vi "MMF with Identical Structure Element.vi"(7 "signal length":i32, 8 "start index":i32, 9 "operation type":u16(ring) items=["Dilation", "Erosion"], 10 "Structure Element":dbl[](array[numeric]), 11 "Extended X":dbl[](array[numeric])) -> (3 "Filtered X":dbl[](array[numeric]))   [LabVIEW 2020, in "NI_AAL_Filter.lvlib"]
uses:
  <vilib>/Analysis/NI_AAL_Filter.lvlib
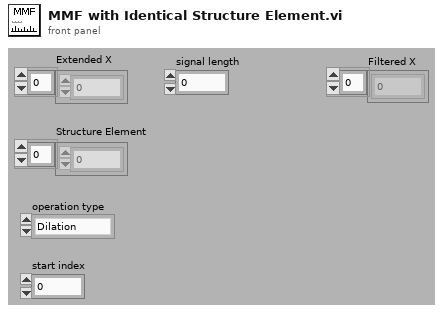
[diagram p1: front panel]
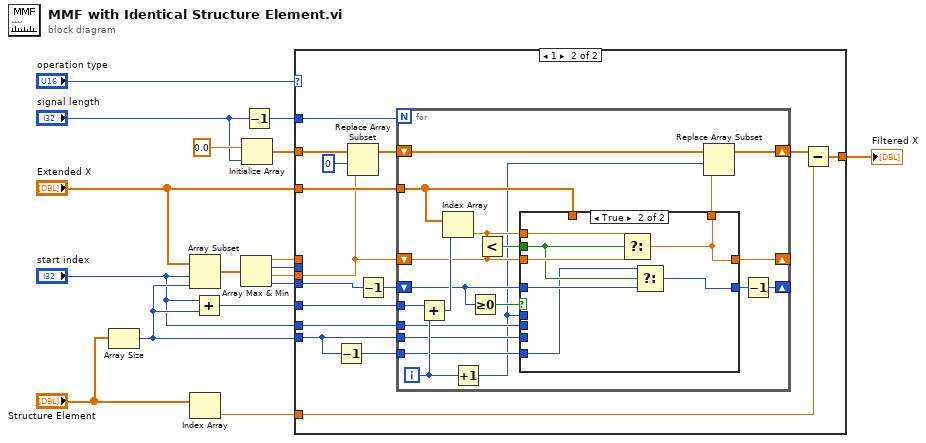
[diagram p0: block diagram]
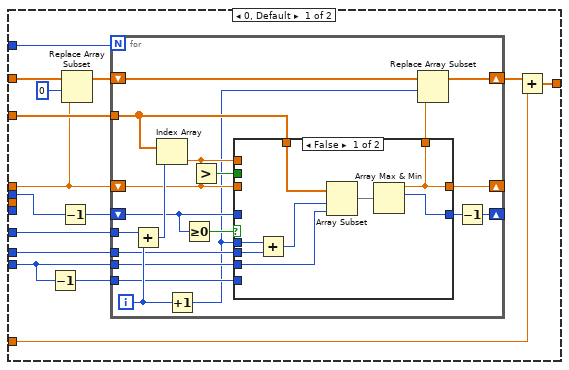
[diagram p2: hidden frame]
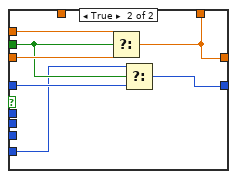
[diagram p3: hidden frame]
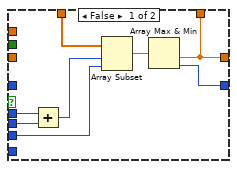
[diagram p4: hidden frame]
diagram:
  n1 = Array Size(array="Structure Element") -> (size(s)=w4:i32)
  n2 = Array Subset(array="Extended X", index="start index", length=w4) -> (w16:dbl[])
  n3 = Index Array(array="Structure Element") -> (element=w10:dbl)  [unwired: 1 in]
  n4 = Add(x="start index", y=w4) -> (x+y=w7:i32)
  n5 = Array Max & Min(array=w16) -> (max value=w11:dbl, max index (indices)=w5:i32, min value=w9:dbl, min index (indices)=w2:i32)
  n6 = Initialize Array(0.0 ("element"), "signal length") -> (w12:dbl[])
  n7 = Decrement(x="signal length") -> (x-1=w13:i32)
  n8 = case shown="1" "operation type" {
    tunnel: w13 -> [w32 w81]
    tunnel: w12 -> [w31 w80]
    tunnel: w11 -> [w26 _]
    tunnel: w10 -> [w24 w74]
    tunnel: w9 -> [_ w68]
    tunnel: "Extended X" -> [w28 w77]
    tunnel: w7 -> [w27 w76]
    tunnel: [w23 w73] -> w6
    tunnel: w5 -> [w22 _]
    tunnel: w4 -> [w20 w71]
    tunnel: "start index" -> [w19 w70]
    tunnel: w2 -> [_ w69]
    frame 0, Default {
      n9 = Decrement(x=w20) -> (x-1=w21:i32)
      n10 = Decrement(x=w22) -> (x-1=w18:i32)
      n11 = Replace Array Subset(array=w31, new element=w26, index=0) -> (w29:dbl[])
      n12 = for {
        N: w32 -> [_]
        shift-right: [w48] -> w25
        shift-left: w29 -> [w49]
        tunnel: w28 -> [w36]
        tunnel: w27 -> [w51]
        shift-right: [w40] -> _
        shift-left: w26 -> [w42]
        shift-right: [w37] -> _
        shift-left: w18 -> [w45]
        tunnel: w21 -> [w39]
        tunnel: w20 -> [w35]
        tunnel: w19 -> [w34]
        i -> [w47]
        n13 = Add(x=w51, y=w47) -> (x+y=w50:i32)
        n14 = Index Array(array=w36, index=w50) -> (element=w43:dbl)
        n15 = Increment(x=w47) -> (x+1=w33:i32)
        n16 = Greater Or Equal To 0?(x=w45) -> (x >= 0?=w46:bool)
        n17 = Greater?(x=w43, y=w42) -> (0:w44:bool)
        n18 = case shown="False" w46 {
          tunnel: w45 -> [_ w62]
          tunnel: w44 -> [_ w63]
          tunnel: w43 -> [_ w66]
          tunnel: w42 -> [_ w65]
          tunnel: [w56 w64] -> w41
          tunnel: [w56 w64] -> w40
          tunnel: w39 -> [_ w61]
          tunnel: [w55 w60] -> w38
          tunnel: w36 -> [w59 _]
          tunnel: w35 -> [w58 _]
          tunnel: w34 -> [w54 _]
          tunnel: w33 -> [w53 _]
          frame False {
            n19 = Add(x=w53, y=w54) -> (x+y=w52:i32)
            n20 = Array Subset(array=w59, index=w52, length=w58) -> (w57:dbl[])
            n21 = Array Max & Min(array=w57) -> (max value=w56:dbl, max index (indices)=w55:i32)  [unwired: 2 out]
          }
          frame True {
            n22 = Select(t=w66, s=w63, f=w65) -> (s? t:f=w64:dbl)
            n23 = Select(t=w61, s=w63, f=w62) -> (s? t:f=w60:i32)
          }
        }
        n24 = Replace Array Subset(array=w49, new element=w41, index=w33) -> (w48:dbl[])
        n25 = Decrement(x=w38) -> (x-1=w37:i32)
      }
      n26 = Add(x=w25, y=w24) -> (x+y=w23:dbl[])
    }
    frame 1 {
      n27 = Decrement(x=w71) -> (x-1=w72:i32)
      n28 = Replace Array Subset(array=w80, new element=w68, index=0) -> (w78:dbl[])
      n29 = Decrement(x=w69) -> (x-1=w67:i32)
      n30 = for {
        N: w81 -> [_]
        shift-right: [w97] -> w75
        shift-left: w78 -> [w98]
        tunnel: w77 -> [w85]
        tunnel: w76 -> [w100]
        shift-right: [w89] -> _
        shift-left: w68 -> [w91]
        shift-right: [w86] -> _
        shift-left: w67 -> [w94]
        tunnel: w72 -> [w88]
        tunnel: w71 -> [w84]
        tunnel: w70 -> [w83]
        i -> [w96]
        n31 = Add(x=w100, y=w96) -> (x+y=w99:i32)
        n32 = Index Array(array=w85, index=w99) -> (element=w92:dbl)
        n33 = Increment(x=w96) -> (x+1=w82:i32)
        n34 = Greater Or Equal To 0?(x=w94) -> (x >= 0?=w95:bool)
        n35 = Less?(x=w92, y=w91) -> (x < y?=w93:bool)
        n36 = case shown="True" w95 {
          tunnel: w94 -> [_ w111]
          tunnel: w93 -> [_ w112]
          tunnel: w92 -> [_ w115]
          tunnel: w91 -> [_ w114]
          tunnel: [w102 w113] -> w90
          tunnel: [w102 w113] -> w89
          tunnel: w88 -> [_ w110]
          tunnel: [w101 w109] -> w87
          tunnel: w85 -> [w108 _]
          tunnel: w84 -> [w107 _]
          tunnel: w83 -> [w105 _]
          tunnel: w82 -> [w104 _]
          frame False {
            n37 = Add(x=w104, y=w105) -> (x+y=w103:i32)
            n38 = Array Subset(array=w108, index=w103, length=w107) -> (w106:dbl[])
            n39 = Array Max & Min(array=w106) -> (min value=w102:dbl, min index (indices)=w101:i32)  [unwired: 2 out]
          }
          frame True {
            n40 = Select(t=w115, s=w112, f=w114) -> (s? t:f=w113:dbl)
            n41 = Select(t=w110, s=w112, f=w111) -> (s? t:f=w109:i32)
          }
        }
        n42 = Replace Array Subset(array=w98, new element=w90, index=w82) -> (w97:dbl[])
        n43 = Decrement(x=w87) -> (x-1=w86:i32)
      }
      n44 = Subtract(x=w75, y=w74) -> (x-y=w73:dbl[])
    }
  }
  "Filtered X" <- w6
